vi "takepressure_2.vi"() -> ()   [LabVIEW 2011]
panel:
  out "Pressure Output":cluster{"Y":dbl[], "Y":dbl[]}[](graph)
  in  "Wait for Shot Event":bool
  in  "Sample Rate":dbl=10.0
  in  "Sampling Time":dbl=60.0
  in  "stop":bool
  out "Shot Number":i32
  in  "Tree":string="machine"
  in  "Start Event":string="Shot_Init"
  out "Connect status":i32
  in  "Host":string="shanghai.ph.utexas.edu"
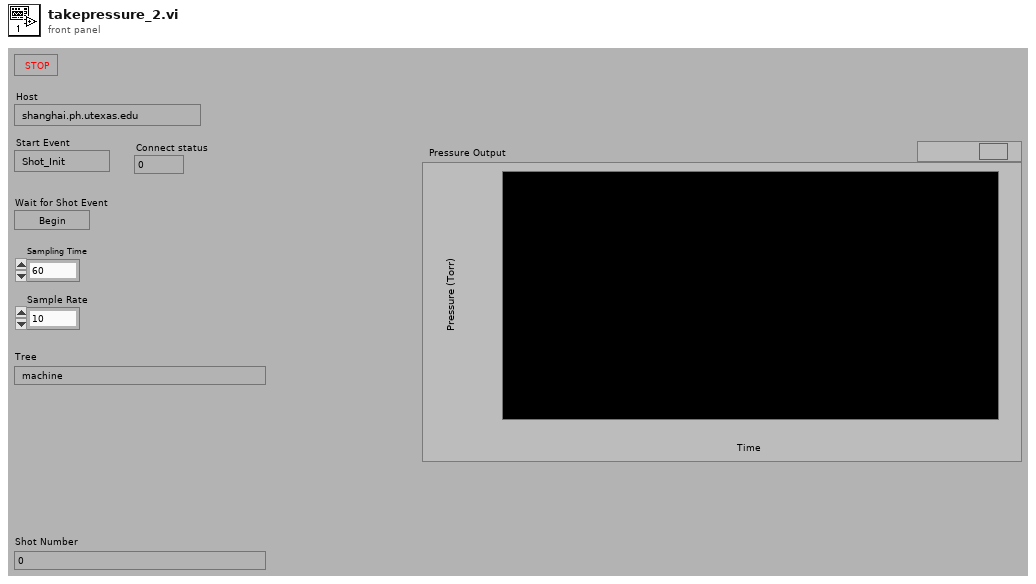
[diagram p1: front panel]
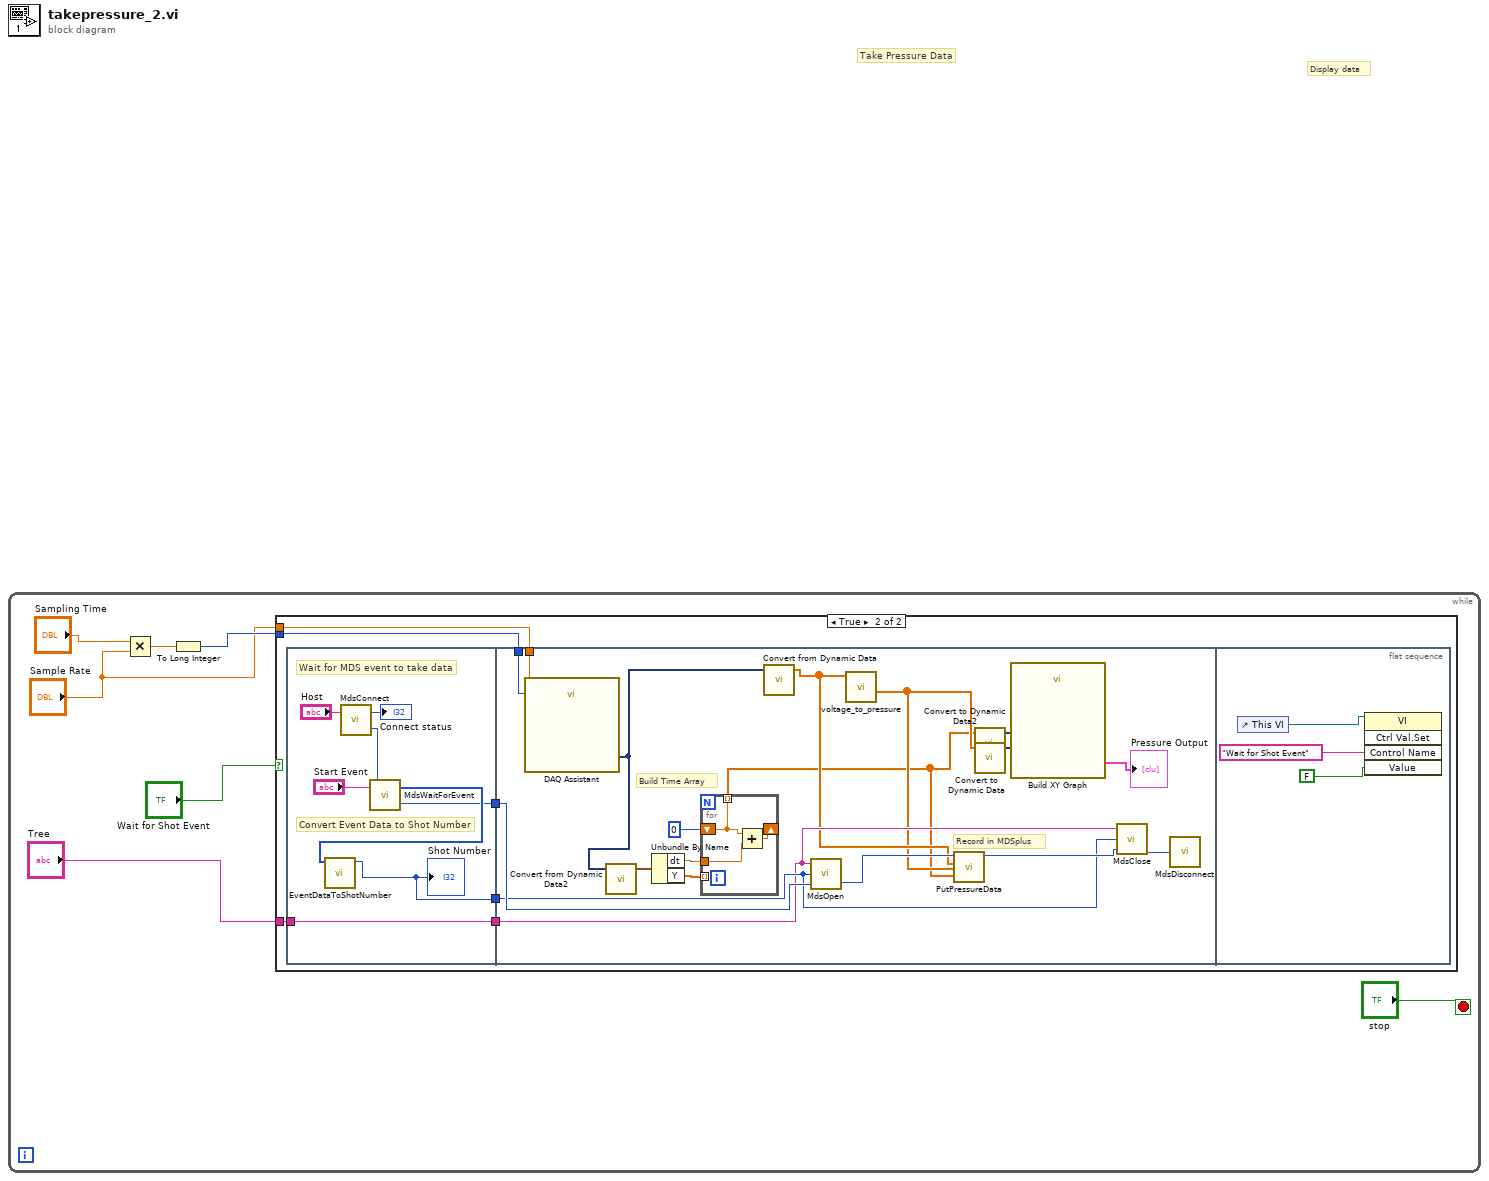
[diagram p0: block diagram]
diagram:
  # "Display data"
  # "Take Pressure Data"
  n1 = while {
    stop <- "stop" stop-if-true
    n2 = Multiply(x="Sampling Time", y="Sample Rate") -> (x*y=w5:dbl)
    n3 = To Long Integer(number=w5) -> (32bit integer=w4:i32)
    n4 = case shown="True" "Wait for Shot Event" {
      tunnel: w4 -> [_ w13]
      tunnel: "Sample Rate" -> [_ w12]
      tunnel: "Tree" -> [_ w8]
      frame False {
      }
      frame True {
        n5 = flat-sequence {
          tunnel: [w16] -> w11
          tunnel: [w15] -> w10
          tunnel: [w14] -> w9
          tunnel: w8 -> [w14]
          tunnel: w13 -> [w40]
          tunnel: w12 -> [w39]
          tunnel: w11 -> [w26]
          tunnel: w10 -> [w32]
          tunnel: w9 -> [w25]
          frame #0 {
            # "Convert Event Data to Shot Number"
            # "Wait for MDS event to take data"
            n6 = call "MdsConnect.vi"("Host"="Host") -> ("FlowControlOut"=w20:i32, "Status"=→"Connect status":i32)  [unwired: 1 in]
            n7 = call "MdsWaitForEvent.vi"("FlowControlIn"=w20, "Event"="Start Event") -> ("FlowControlOut"=w15:i32, "EventData"=w21:u8[])
            n8 = call "EventDataToShotNumber.vi"("EventDataIn"=w21) -> ("ShotNumberOut"=w16:i32)  [unwired: 10 in]
            "Shot Number" <- w16
          }
          frame #1 {
            # "Record in MDSplus"
            # "Build Time Array"
            n9 = call "DAQ Assistant"("rate"=w39, "number of samples"=w40) -> ("data"=w34:dynamicdata)  [unwired: 15 in, 2 out]
            n10 = call "Convert from Dynamic Data2"("Dynamic Data Type"=w34) -> ("Waveform"=w36:waveform(dbl))  [unwired: 3 in]
            n11 = Unbundle By Name(w36) -> ("dt"=w37:dbl, "Y"=w38:dbl[])
            n12 = for {
              shift-right: [w42] -> _
              shift-left: 0 -> [w41]
              tunnel: w37 -> [w43]
              tunnel: [w41] -> w22 mode=indexing
              tunnel: w38 -> [_] mode=indexing
              n13 = Add(x=w41, y=w43) -> (x+y=w42:dbl)
            }
            n14 = call "Convert from Dynamic Data"("Dynamic Data Type"=w34) -> ("Array"=w24:dbl[])  [unwired: 3 in]
            n15 = call "MdsOpen.vi"("FlowControlIn"=w32, "Shot"=w26, "Tree"=w25) -> ("FlowControlOut"=w28:i32)  [unwired: 1 out]
            n16 = call "voltage_to_pressure.vi"("Voltage In"=w24) -> ("Pressure Out"=w23:dbl[])  [unwired: 8 in, 2 out]
            n17 = call "PutPressureData.vi"("Time"=w22, "Pressure"=w23, "Voltage"=w24, "FlowControlIn"=w28) -> ("FlowControlOut"=w27:i32)  [unwired: 7 in]
            n18 = call "Convert to Dynamic Data2"("Array"=w22) -> ("Dynamic Data Type"=w29:dynamicdata)  [unwired: 3 in]
            n19 = call "Convert to Dynamic Data"("Array"=w23) -> ("Dynamic Data Type"=w30:dynamicdata)  [unwired: 3 in]
            n20 = call "Build XY Graph"("Y Input"=w30, "X Input"=w29) -> ("XY Graph"=→"Pressure Output":cluster{"Y":dbl[], "Y":dbl[]}[])  [unwired: 3 in, 6 out]
            n21 = call "MdsClose.vi"("FlowControlIn"=w27, "Shot"=w26, "Tree"=w25) -> ("FlowControlOut"=w33:i32)  [unwired: 1 out]
            n22 = call "MdsDisconnect.vi"("FlowControlIn"=w33) -> ()  [unwired: 1 out]
          }
          frame #2 {
            n23 = control-ref of="This VI"() -> (w45:refnum<vi>)
            n24 = invoke class="VI" method="Ctrl Val.Set"(reference=w45, "Control Name"="Wait for Shot Event", "Value"=FALSE) -> ()  [unwired: 2 in, 5 out]
          }
        }
      }
    }
  }
